vi "Error Source Overwrite.vi"(5 "always (F)":bool, 6 "error in":errorcluster, 7 "append time (T)":bool=TRUE, 9 "source":string="New source.") -> (0 "error out":errorcluster)   [LabVIEW 2020]
doc: "This function overwrites the error cluster source field, with an option to append the current time. The error cluster status and code fields are unchanged."
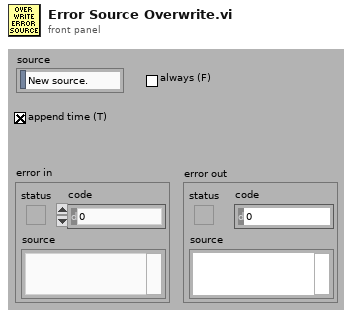
[diagram p1: front panel]
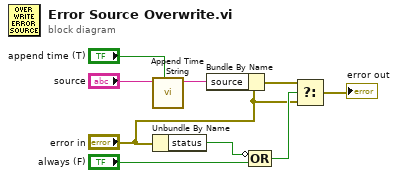
[diagram p0: block diagram]
diagram:
  n1 = call "Append Time String.vi"("enable (T)"="append time (T)", "string in"="source") -> ("string out"=w3:string)  [unwired: 5 in, 1 out]
  n2 = Unbundle By Name("error in") -> ("status"=w6:bool)
  n3 = Bundle By Name(cluster="error in", "source"=w3) -> (w2:errorcluster)
  n4 = Compound Arithmetic op=OR(invert w6, "always (F)") -> (w9:bool)
  n5 = Select(t=w2, s=w9, f="error in") -> (s? t:f=→"error out":errorcluster)
